vi "CPID Engine.vi"(8 "error in":errorcluster, 11 "State Variables":T1={"TCP Refs"={"Connection List"=refnum, "listener ID"=refnum}, "Stop"=refnum, "Top VI"=refnum, "Parameters"={"Name"="", "PID Lookup"=variant, "DID Lookup"=variant, "Section Properties"={"CAN"={"Database File"=path "", "CAN Interface"=enum."CAN0", "Baud Rate"=0, "Diagnostic Protocol"=enum."GMLAN", "Transport Protocol"=enum."ISO TP - Normal Mode", "Transmit ID"=0, "Receive ID"=0, "Transmit Extension"=0, "Receive Extension"=0, "Receive UUDT ID"=0, "Enable Stream"=TRUE, "VW TP Channel ID"=0}, "DPIDs"=[], "DTC descriptor"={"DTC Byte Length"=2, "Status Byte Length"=1, "Add Data Byte Length"=1, "Byte Order"=enum."Motorola"}, "PIDs"=[], "DIDs"=[], "CPIDs"=[]}, "ChanRefs"={"ToVS.PIDs"={"Name"="", "Write to VS Engine FIFO"=refnum, "Pairs"={"Refs"=[], "Values"=[]}}, "ToVS.DIDs"={"Name"="", "Write to VS Engine FIFO"=refnum, "Pairs"={"Refs"=[], "Values"=[]}}, "ToVS.DTCs"={"Name"="", "Write to VS Engine FIFO"=refnum, "Pairs"={"Refs"=[], "Values"=[]}}, "ToVS.DTCCount"={"Name"="", "Write to VS Engine FIFO"=refnum, "Pairs"={"Refs"=[], "Values"=[]}}, "ToVS.Success"={"Name"="", "Write to VS Engine FIFO"=refnum, "Pairs"={"Refs"=[], "Values"=[]}}, "FromVS.CPIDs"={"Name"="", "Read from VS Engine FIFO"=refnum, "Pairs"={"Refs"=[], "Values"=[]}}, "Cmds"={"Name"="", "Write to VS Engine FIFO"=refnum, "Read from VS Engine FIFO"=refnum, "Pairs"={"Chan Refs"=[], "Prev. Values"=[]}}}, "CPID Lookup"=variant, "DPID Lookup"=variant}, "ADCS Connection"={"Diag CAN Handle"=0, "Transport Protocol"=enum."ISO TP - Normal Mode", "Receive Address Extension"=0, "Transmit Address Extension"=0, "Receive CAN Id"=0, "Transmit CAN Id"=0, "Diag CAN Queue"=refnum, "Log Frames ?"=FALSE, "My TP Address"=0, "Other TP Address"=0, "T1"=0, "T2"=0, "T3"=0, "T4"=0, "Tx SN"=0, "Block Size"=0, "Rx SN"=0, "VW TP Initialized?"=FALSE, "Tx block no"=0, "baud rate"=0, "Interface"="", "Channel Diag CAN Handle"=0, "UDP Connection ID"=refnum, "TCP Connection ID"=refnum, "Target IP Addr"=0, "Source Address"=0, "Target Address"=0, "Send Header NACK?"=FALSE, "DLL Handle"=0, "NAD"=0}, "XNET References"={"Database"="", "GMLAN DPID Session"="", "Cluster"=""}, "BufferedCmds"=refnum, "XNETEngine (GMLAN)"=refnum} {"Parameters"."ChanRefs"."Cmds"."Pairs"."Chan Refs" format="%.0x"; "Parameters"."ChanRefs"."ToVS.Success"."Pairs"."Refs" format="%.0x"; "Parameters"."ChanRefs"."ToVS.DTCCount"."Pairs"."Refs" format="%.0x"; "Parameters"."ChanRefs"."ToVS.DTCs"."Pairs"."Refs" format="%.0x"; "Parameters"."ChanRefs"."ToVS.PIDs"."Pairs"."Refs" format="%.0x"; "Parameters"."ChanRefs"."ToVS.DIDs"."Pairs"."Refs" format="%.0x"; "Parameters"."Section Properties"."CPIDs"."Signals"."Byte Order" items=["Little Endian", "Big Endian"]; "Parameters"."Section Properties"."CPIDs"."Signals"."Data Type" items=["Signed", "Unsigned", "IEEE Float"]; "Parameters"."Section Properties"."DIDs"."Signals"."Byte Order" items=["Little Endian", "Big Endian"]; "Parameters"."Section Properties"."DIDs"."Signals"."Data Type" items=["Signed", "Unsigned", "IEEE Float"]; "Parameters"."Section Properties"."CAN"."VW TP Channel ID" format="%.0x"; "Parameters"."Section Properties"."CAN"."Receive UUDT ID" format="%.0x"; "Parameters"."Section Properties"."CAN"."Receive Extension" format="%.0x"; "Parameters"."Section Properties"."CAN"."Transmit Extension" format="%.0x"; "Parameters"."Section Properties"."CAN"."Receive ID" format="%.0x"; "Parameters"."Section Properties"."CAN"."Transmit ID" format="%.0x"; "Parameters"."Section Properties"."PIDs"."Signals"."Byte Order" items=["Little Endian", "Big Endian"]; "Parameters"."Section Properties"."PIDs"."Signals"."Data Type" items=["Signed", "Unsigned", "IEEE Float"]}) -> (0 "error out":errorcluster)   [LabVIEW 2013, in "Diagnostics Addon Engine.lvlib"]
uses:
  Diagnostics Addon Engine.lvlib
  State Variables.ctl
  TCP Refs.ctl
  STM/STM Lookup Table Ref.ctl
  Stop FG/Stop Global Ref.ctl
  Main Configuration.ctl
  Section Properties.ctl
  Shared/CAN Configuration.ctl
  Shared/CAN Interface.ctl
  Shared/Diagnostic Protocols.ctl
  Shared/Transport Protocols.ctl
  Shared/DPID Parameters.ctl
  Shared/DPID Periodic Rate.ctl
  <vilib>/Automotive Diagnostic Command Set/Diagnostic Protocols.llb/DTC Descriptor.ctl
  Shared/DIDPID Parameters.ctl
  Shared/DIDPID Signal Parameters.ctl
  VS Data Channels.ctl
  Inline Async API/Controls/Write To VS Engine.ctl
  <vilib>/NI Veristand/Custom Device API/Data Reference.ctl
  Inline Async API/Controls/Read From VS Engine.ctl
  <vilib>/NI Veristand/Custom Device API/Block Data Reference.ctl
  Inline Async API/Controls/ReadWrite Data.ctl
  <vilib>/Automotive Diagnostic Command Set/Diagnostic Transport.llb/Diag Reference.ctl
  <vilib>/Automotive Diagnostic Command Set/Diagnostic Transport.llb/Transport Protocol Selector.ctl
  <vilib>/Automotive Diagnostic Command Set/Diagnostic Transport.llb/Diag CAN Frame Log.ctl
  XNET References.ctl
  <vilib>/NI/AMC/Message Queue.ctl
  <vilib>/NI/AMC/Message.ctl
  <vilib>/NI/Tools/Keyed Array/KeyedArray.ctl
  Stop FG/Stop Global Commands.ctl
  Datatable Lookup Positions.ctl
  CPID Conversion Cluster.ctl
  <vilib>/NI/AMC/Create Single Message.vi
  <vilib>/NI/AMC/Update Message Routing Info.vi
  Shared/GUID Lookup.vi
  <vilib>/xnet/xnet.llb/XNET Convert (Signal to Frame Raw).vi
  <vilib>/NI/AMC/Send Message.vi
  Error Handling API/Error Handling API.lvlib
  Shared/Diagnostics Addon Shared.lvlib
  <vilib>/NI Veristand/Custom Device Tools/Custom Device Utility Library/Custom Device Utility Library.lvlib
  Stop FG/Stop FG.lvlib
  <vilib>/NI/AMC/AMC.lvlib
  <vilib>/NI Veristand/Custom Device API/Custom Device API.lvlib
  <vilib>/NI/Tools/Keyed Array/Tools_KeyedArray.lvlib
  <vilib>/addons/Automotive Diagnostic Command Set/NI_Automotive Diagnostic Command Set.lvlib
  Inline Async API/Inline Async API.lvlib
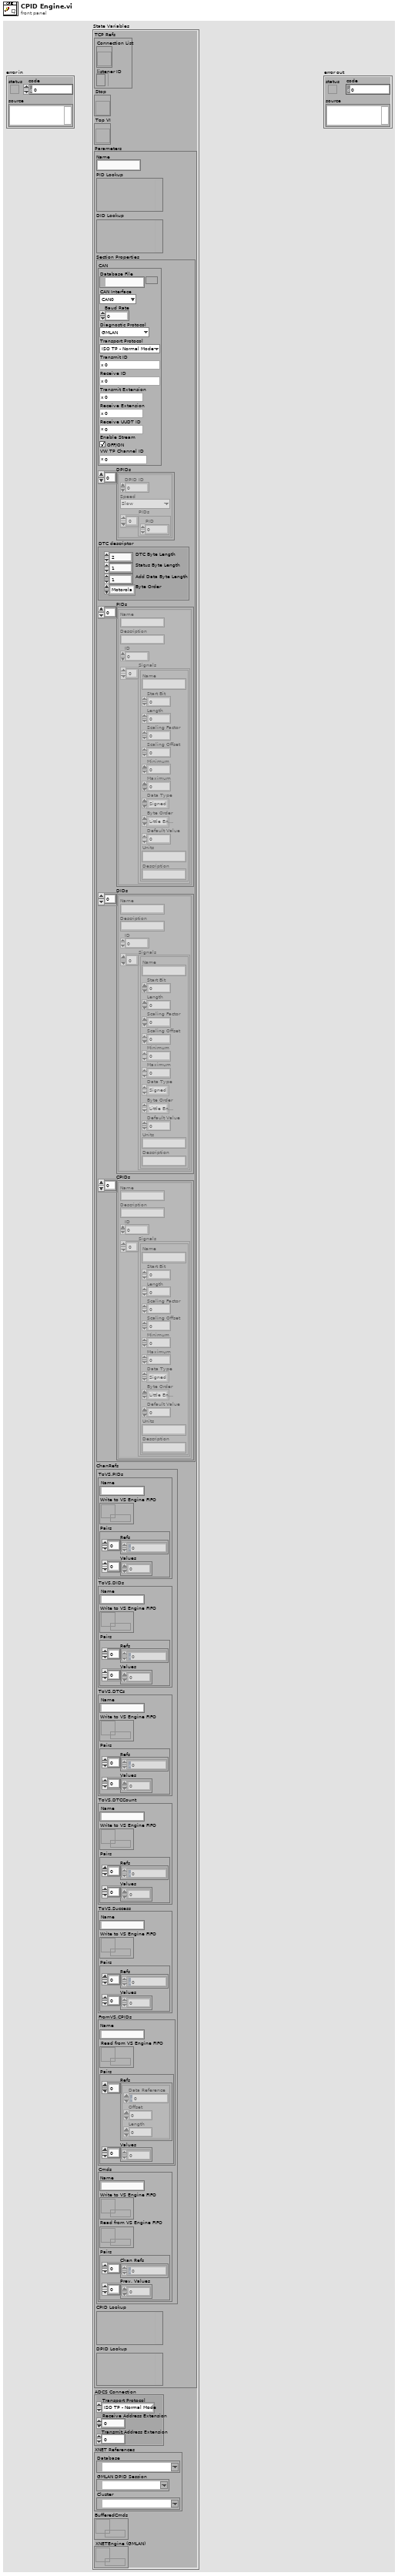
[diagram p1: front panel]
types:
  T1 = typedef "Diagnostics Addon Engine.lvlib/State Variables.ctl" = cluster{"TCP Refs":T2, "Stop":T4, "Top VI":refnum<vi>, "Parameters":T5, "ADCS Connection":T22, "XNET References":T24, "BufferedCmds":T25, "XNETEngine (GMLAN)":T25}
  T2 = typedef "Diagnostics Addon Engine.lvlib/TCP Refs.ctl" = cluster{"Connection List":T3, "listener ID":refnum<k5>}
  T3 = typedef "Diagnostics Addon Engine.lvlib/STM Lookup Table Ref.ctl" = refnum<vi>
  T4 = typedef "Diagnostics Addon Engine.lvlib/Stop FG.lvlib/Stop Global Ref.ctl" = refnum<vi>
  T5 = typedef "Diagnostics Addon Engine.lvlib/Main Configuration.ctl" = cluster{"Name":string, "PID Lookup":variant, "DID Lookup":variant, "Section Properties":T6, "ChanRefs":T16, "CPID Lookup":variant, "DPID Lookup":variant}
  T6 = typedef "Diagnostics Addon Engine.lvlib/Section Properties.ctl" = cluster{"CAN":T7, "DPIDs":T11[], "DTC descriptor":T13, "PIDs":T14[], "DIDs":T14[], "CPIDs":T14[]}
  T7 = typedef "Diagnostics Addon Shared.lvlib/CAN Configuration.ctl" = cluster{"Database File":path, "CAN Interface":T8, "Baud Rate":u32, "Diagnostic Protocol":T9, "Transport Protocol":T10, "Transmit ID":u32, "Receive ID":u32, "Transmit Extension":u8, "Receive Extension":u8, "Receive UUDT ID":u32, "Enable Stream":bool, "VW TP Channel ID":u32}
  T8 = typedef "Diagnostics Addon Shared.lvlib/CAN Interface.ctl" = enum16{"CAN0", "CAN1", "CAN2", "CAN3", "CAN4", "CAN5", "CAN6", "CAN7", "CAN8", "CAN9", "CAN10", "CAN11", "CAN12", "CAN13", "CAN14", "CAN15", "CAN16", "CAN17", "CAN18", "CAN19", "CAN20", "CAN21", "CAN22", "CAN23", "CAN24", "CAN25", "CAN26", "CAN27", "CAN28", "CAN29", "CAN30", "CAN31", "CAN32", "CAN33", "CAN34", "CAN35", "CAN36", "CAN37", "CAN38", "CAN39", "CAN40", "CAN41", "CAN42", "CAN43", "CAN44", "CAN45", "CAN46", "CAN47", "CAN48", "CAN49", "CAN50", "CAN51", "CAN52", "CAN53", "CAN54", "CAN55", "CAN56", "CAN57", "CAN58", "CAN59", "CAN60", "CAN61", "CAN62", "CAN63", "CAN 256 (Virtual)", "CAN 257 (Virtual)"}
  T9 = typedef "Diagnostics Addon Shared.lvlib/Diagnostic Protocols.ctl" = enum16{"GMLAN", "KWP-2000", "UDS"}
  T10 = typedef "Diagnostics Addon Shared.lvlib/Transport Protocols.ctl" = enum16{"ISO TP - Normal Mode", "ISO TP - Mixed Mode", "VW TP 2.0", "Diagnostics on IP"}
  T11 = typedef "Diagnostics Addon Shared.lvlib/DPID Parameters.ctl" = cluster{"DPID ID":u8, "Speed":T12, "PIDs":u16[]}
  T12 = typedef "Diagnostics Addon Shared.lvlib/DPID Periodic Rate.ctl" = enum16{"Slow", "Medium", "Fast"}
  T13 = typedef "DTC Descriptor.ctl" = cluster{"DTC Byte Length":i32, "Status Byte Length":i32, "Add Data Byte Length":i32, "Byte Order":enum16{"Motorola", "Intel"}}
  T14 = typedef "Diagnostics Addon Shared.lvlib/DIDPID Parameters.ctl" = cluster{"Name":string, "Description":string, "ID":u16, "Signals":T15[]}
  T15 = typedef "Diagnostics Addon Shared.lvlib/DIDPID Signal Parameters.ctl" = cluster{"Name":string, "Start Bit":u8, "Length":u8, "Scaling Factor":dbl, "Scaling Offset":dbl, "Minimum":dbl, "Maximum":dbl, "Data Type":u32, "Byte Order":u32, "Default Value":dbl, "Units":string, "Description":string}
  T16 = typedef "Diagnostics Addon Engine.lvlib/VS Data Channels.ctl" = cluster{"ToVS.PIDs":T17, "ToVS.DIDs":T17, "ToVS.DTCs":T17, "ToVS.DTCCount":T17, "ToVS.Success":T17, "FromVS.CPIDs":T19, "Cmds":T21}
  T17 = typedef "Diagnostics Addon Engine.lvlib/Inline Async API.lvlib/Write To VS Engine.ctl" = cluster{"Name":string, "Write to VS Engine FIFO":refnum<k33>, "Pairs":cluster{"Refs":T18[], "Values":dbl[]}}
  T18 = typedef "Custom Device API.lvlib/Data Reference.ctl" = i32
  T19 = typedef "Diagnostics Addon Engine.lvlib/Inline Async API.lvlib/Read From VS Engine.ctl" = cluster{"Name":string, "Read from VS Engine FIFO":refnum<k33>, "Pairs":cluster{"Refs":T20[], "Values":dbl[]}}
  T20 = typedef "Custom Device API.lvlib/Block Data Reference.ctl" = cluster{"Data Reference":T18, "Offset":i32, "Length":i32}
  T21 = typedef "Diagnostics Addon Engine.lvlib/Inline Async API.lvlib/ReadWrite Data.ctl" = cluster{"Name":string, "Write to VS Engine FIFO":refnum<k33>, "Read from VS Engine FIFO":refnum<k33>, "Pairs":cluster{"Chan Refs":T18[], "Prev. Values":dbl[]}}
  T22 = typedef "NI_Automotive Diagnostic Command Set.lvlib/Diag Reference.ctl" = cluster{"Diag CAN Handle":u32, "Transport Protocol":T23, "Receive Address Extension":u8, "Transmit Address Extension":u8, "Receive CAN Id":u32, "Transmit CAN Id":u32, "Diag CAN Queue":refnum<queue>, "Log Frames ?":bool, "My TP Address":u8, "Other TP Address":u8, "T1":u16, "T2":u16, "T3":u16, "T4":u16, "Tx SN":u8, "Block Size":u8, "Rx SN":u8, "VW TP Initialized?":bool, "Tx block no":u8, "baud rate":u32, "Interface":string, "Channel Diag CAN Handle":u32, "UDP Connection ID":refnum<k16>, "TCP Connection ID":refnum<k5>, "Target IP Addr":u32, "Source Address":u16, "Target Address":u16, "Send Header NACK?":bool, "DLL Handle":u32, "NAD":u8}
  T23 = typedef "NI_Automotive Diagnostic Command Set.lvlib/Transport Protocol Selector.ctl" = enum16{"ISO TP - Normal Mode", "ISO TP - Mixed Mode", "VW TP 2.0", "Diagnostics on IP", "ISO TP LIN"}
  T24 = typedef "Diagnostics Addon Engine.lvlib/XNET References.ctl" = cluster{"Database":refnum<k21>, "GMLAN DPID Session":refnum<k21>, "Cluster":refnum<k21>}
  T25 = typedef "AMC.lvlib/Message Queue.ctl" = refnum<queue>
  T26 = typedef "Diagnostics Addon Engine.lvlib/CPID Conversion Cluster.ctl" = cluster{"ID":u16, "Position":T27, "Conversion":refnum<k21>, "Frame Length":u8}
  T27 = typedef "Diagnostics Addon Engine.lvlib/Datatable Lookup Positions.ctl" = cluster{"Offset":i32, "Length":i32}
  T28 = typedef "Diagnostics Addon Engine.lvlib/Stop FG.lvlib/Stop Global Commands.ctl" = enum16{"Write", "Read", "Reset"}
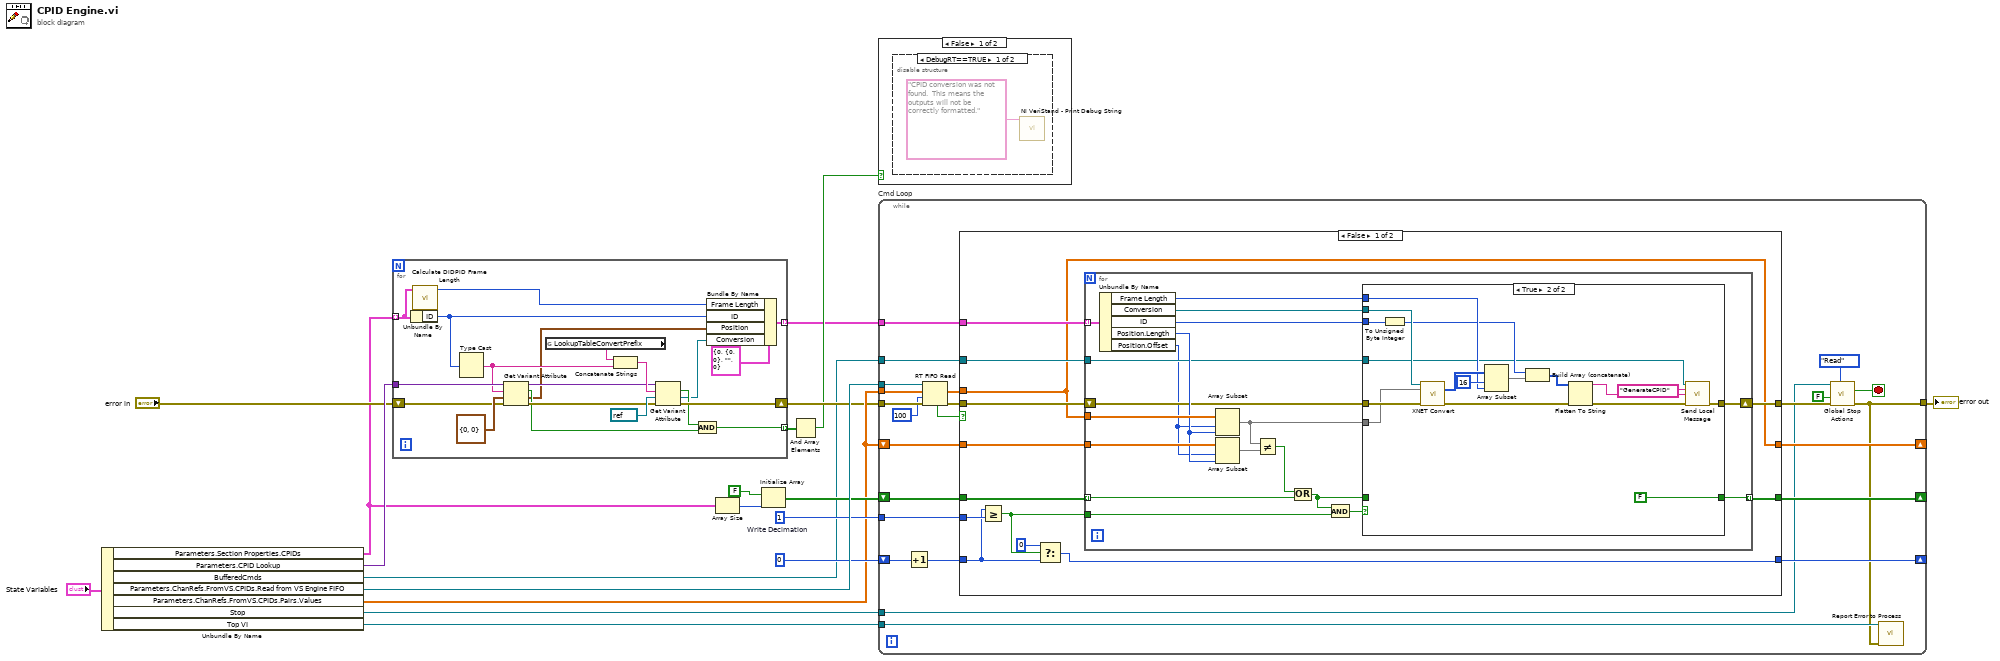
[diagram p0: block diagram]
diagram:
  w14 = u32 1  # Write Decimation
  n1 = Unbundle By Name("State Variables") -> ("Parameters.Section Properties.CPIDs"=w5:T14[], "Parameters.CPID Lookup"=w9:variant, "BufferedCmds"=w6:T25, "Parameters.ChanRefs.FromVS.CPIDs.Read from VS Engine FIFO"=w18:refnum<k33>, "Parameters.ChanRefs.FromVS.CPIDs.Pairs.Values"=w10:dbl[], "Stop"=w12:T4, "Top VI"=w11:refnum<vi>)
  n2 = for {
    tunnel: w5 -> [w21] mode=indexing
    tunnel: w9 -> [w39]
    shift-right: [w32] -> w7
    shift-left: "error in" -> [w37]
    tunnel: [w27] -> w4 mode=indexing
    tunnel: [w24] -> w1 mode=indexing
    n3 = Unbundle By Name(w21) -> ("ID"=w26:u16)
    n4 = call "Calculate DIDPID Frame Length.vi"("PID In"=w21) -> ("Frame Length"=w20:u8)  [unwired: 10 in]
    n5 = Type Cast(x=w26) -> (*(type *) &x=w31:string)  [unwired: 1 in]
    n6 = Get Variant Attribute(Variant=w39, name=w31, default value (empty Variant)=T27 {"Offset"=0, "Length"=0} ("cluster"), error in=w37) -> (duplicate Variant=w30:variant, found=w28:bool, value=w23:T27, error out=w33:errorcluster)
    n7 = global read "GUID Lookup.vi" "LookupTableConvertPrefix"() -> (w34:string)
    n8 = Concatenate Strings(w34, w31) -> (w35:string)
    n9 = Get Variant Attribute(Variant=w30, name=w35, default value (empty Variant)=refnum<k21> refnum ("DID Conversion"), error in=w33) -> (found=w29:bool, value=w22:refnum<k21>, error out=w32:errorcluster)  [unwired: 1 out]
    n10 = Compound Arithmetic op=AND(w29, w28) -> (w27:bool)
    n11 = Bundle By Name(cluster=T26 {"ID"=0, "Position"={"Offset"=0, "Length"=0}, "Conversion"="", "Frame Length"=0}, "Frame Length"=w20, "ID"=w26, "Position"=w23, "Conversion"=w22) -> (w24:T26)
  }
  n12 = Array Size(array=w5) -> (size(s)=w16:i32)
  n13 = Initialize Array(FALSE, w16) -> (w15:bool[])
  n14 = And Array Elements(Boolean array=w4) -> (logical AND=w3:bool)
  n15 = case shown="False" w3 {
    frame False {
      n16 = disable-structure shown="DebugRT==TRUE" {
        frame condition #0 {
          n17 = call <vilib>:"NI VeriStand - Print Debug String.vi"("Message"="CPID conversion was not found.  This means the outputs will not be correctly formatted." ("Debug String")) -> ()  [unwired: 10 in, 1 out]
        }
        frame condition #1 (active) {
        }
      }
    }
    frame True {
    }
  }
  n18 = while "Cmd Loop" {
    tunnel: w7 -> [w64]
    tunnel: [w41] -> w2
    tunnel: w18 -> [w63]
    shift-right: [w54] -> _
    shift-left: 0 ("t") -> [w56]
    shift-right: [w59] -> _
    shift-left: w15 -> [w58]
    tunnel: w14 -> [w57]
    tunnel: w12 -> [w45]
    tunnel: w11 -> [w52]
    tunnel: w10 -> [w51]
    shift-right: [w49] -> _
    shift-left: w10 -> [w50]
    tunnel: w1 -> [w48]
    tunnel: w6 -> [w47]
    stop <- w42 stop-if-true
    n19 = Increment(x=w56) -> (x+1=w55:i32)
    n20 = RT FIFO Read(0:w63, 1:w51, 2:100 ("timeout in ms (0)"), 3:w64) -> (9:w61:dbl[], 10:w53:bool, 11:w62:errorcluster)  [unwired: 2 out]
    n21 = case shown="False" w53 {
      tunnel: w62 -> [w69 w119]
      tunnel: w61 -> [w65 _]
      tunnel: [w77 w119] -> w46
      tunnel: [w76 w118] -> w59
      tunnel: w58 -> [w75 w118]
      tunnel: w57 -> [w74 _]
      tunnel: w55 -> [w72 w117]
      tunnel: [w70 w117] -> w54
      tunnel: [w65 w116] -> w49
      tunnel: w50 -> [w68 w116]
      tunnel: w48 -> [w67 _]
      tunnel: w47 -> [w66 _]
      frame False {
        n22 = Greater Or Equal?(x=w72, y=w74) -> (x >= y?=w73:bool)
        n23 = Select(t=0, s=w73, f=w72) -> (s? t:f=w70:i32)
        n24 = for {
          tunnel: w68 -> [w96]
          tunnel: w65 -> [w95]
          shift-right: [w92] -> w77
          shift-left: w69 -> [w93]
          tunnel: [w91] -> w76 mode=indexing
          tunnel: w75 -> [w88] mode=indexing
          tunnel: w73 -> [w89]
          tunnel: w67 -> [w84] mode=indexing
          tunnel: w66 -> [w80]
          n25 = Unbundle By Name(w84) -> ("Frame Length"=w79:u8, "Conversion"=w81:refnum<k21>, "ID"=w82:u16, "Position.Length"=w94:i32, "Position.Offset"=w78:i32)
          n26 = Array Subset(array=w95, index=w78, length=w94) -> (w83:dbl[])
          n27 = Array Subset(array=w96, index=w78, length=w94) -> (w85:dbl[])
          n28 = Not Equal?(x=w83, y=w85) -> (x != y?=w87:bool)
          n29 = Or(x=w87, y=w88) -> (x .or. y?=w86:bool)
          n30 = Compound Arithmetic op=AND(w86, w89) -> (w90:bool)
          n31 = case shown="True" w90 {
            tunnel: w93 -> [w98 w113]
            tunnel: [w98 w115] -> w92
            tunnel: [w97 FALSE] -> w91
            tunnel: w86 -> [w97 _]
            tunnel: w83 -> [_ w104]
            tunnel: w82 -> [_ w103]
            tunnel: w81 -> [_ w112]
            tunnel: w80 -> [_ w99]
            tunnel: w79 -> [_ w105]
            frame False {
            }
            frame True {
              n32 = To Unsigned Byte Integer(number=w103) -> (unsigned 8bit integer=w100:u8)
              n33 = call-poly <vilib>:"XNET Convert.vi"("session in"=w112, "signal data"=w104, "error in (no error)"=w113) -> ("frame data"=w111:u8[], "error out"=w109:errorcluster)  [unwired: 10 in, 1 out]
              n34 = Array Subset(array=w111, index=16, length=w105) -> (w102:u8[])
              n35 = Build Array (concatenate)(w100, w102) -> (w101:u8[])
              n36 = Flatten To String(anything=w101, error in (no error)=w109) -> (data string=w107:string, error out=w108:errorcluster)  [unwired: 2 in, 1 out]
              n37 = call <vilib>:"Send Local Message.vi"("message queue in"=w99, "message name"="GenerateCPID" ("Message Name"), "message value"=w107, "error in"=w108) -> ("error out"=w115:errorcluster)  [unwired: 9 in, 2 out]
            }
          }
        }
      }
      frame True {
      }
    }
    n38 = call "Global Stop Actions.vi"("Command"=Stop_Global_Commands."Read", "error in (no error)"=w46, "Stop on Error?"=FALSE, "vi reference"=w45) -> ("error out"=w41:errorcluster, "Latched Stop"=w42:bool)  [unwired: 5 in, 1 out]
    n39 = call "Report Error to Process.vi"("Error"=w41, "This VI"=w52) -> ()  [unwired: 10 in]
  }
  "error out" <- w2
